vi "Stop Core.vi"(10 "final error code":i32, 11 "LF2R IDE in":refnum<class "Main Panel.lvclass">) -> (3 "LF2R IDE out":refnum<class "Main Panel.lvclass">)   [LabVIEW 2018, in "Main Panel.lvlib" / "Main Panel.lvclass"]
doc: "In addition to the following, this method also sends a message to the monitor to notify it that the actor has stopped execution.\n\n(<B>Filename</B>: Actor Framework.lvlib:Actor.lvclass:Stop Core.vi)\n\nDefines what the actor does before it stops. Use the <B>final error code</B> input to determine whether the actor shut down in response to an error.\n\nBy default, this method does nothing. A descendant class may override it to define behavior, such as shutting down any processes the actor initiated in its override of the Actor Core method.\n\nCopyright: MGI\n\nAuthored by Derek Trepanier\nsupport@mooregoodideas.com\nwww.mooregoodideas.com\n\nCopyright (c) 2014, Moore Good Ideas, Inc.\n\nAll rights reserved.\n\nRedistribution and use in source and binary forms, with or without modification, are permitted provided that the following conditions are met:\n\n * Redistributions of source code must retain the above copyright notice, this list of conditions and the following disclaimer.\n * Redistributions in binary form must reproduce the above copyright notice, this list of conditions and the following disclaimer in the documentation and/or other materials provided with the distribution.\n * Neither the name of Moore Good Ideas, Inc. nor the names of its contributors may be used to endorse or promote products derived from this software without specific prior written permission.\n\nTHIS SOFTWARE IS PROVIDED BY THE COPYRIGHT HOLDERS AND CONTRIBUTORS \"AS IS\" AND ANY EXPRESS OR IMPLIED WARRANTIES, INCLUDING, BUT NOT LIMITED TO, THE IMPLIED WARRANTIES OF MERCHANTABILITY AND FITNESS FOR A PARTICULAR PURPOSE ARE DISCLAIMED. IN NO EVENT SHALL THE COPYRIGHT OWNER OR CONTRIBUTORS BE LIABLE FOR ANY DIRECT, INDIRECT, INCIDENTAL, SPECIAL, EXEMPLARY, OR CONSEQUENTIAL DAMAGES (INCLUDING, BUT NOT LIMITED TO, PROCUREMENT OF SUBSTITUTE GOODS OR SERVICES; LOSS OF USE, DATA, OR PROFITS; OR BUSINESS INTERRUPTION) HOWEVER CAUSED AND ON ANY THEORY OF LIABILITY, WHETHER IN CONTRACT, STRICT LIABILITY, OR TORT (INCLUDING NEGLIGENCE OR OTHERWISE) ARISING IN ANY WAY OUT OF THE USE OF THIS SOFTWARE, EVEN IF ADVISED OF THE POSSIBILITY OF SUCH DAMAGE."
uses:
  Main Panel.lvclass
  Main Panel.lvclass/Main Panel.ctl
  Framework/Framework/Framework.lvclass
  <userlib>/_MGI/Menu Building/MenuTypes/Vi/MGI_VI.lvclass
  ScintillaNET/ScintillaNET.lvclass
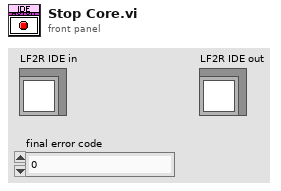
[diagram p1: front panel]
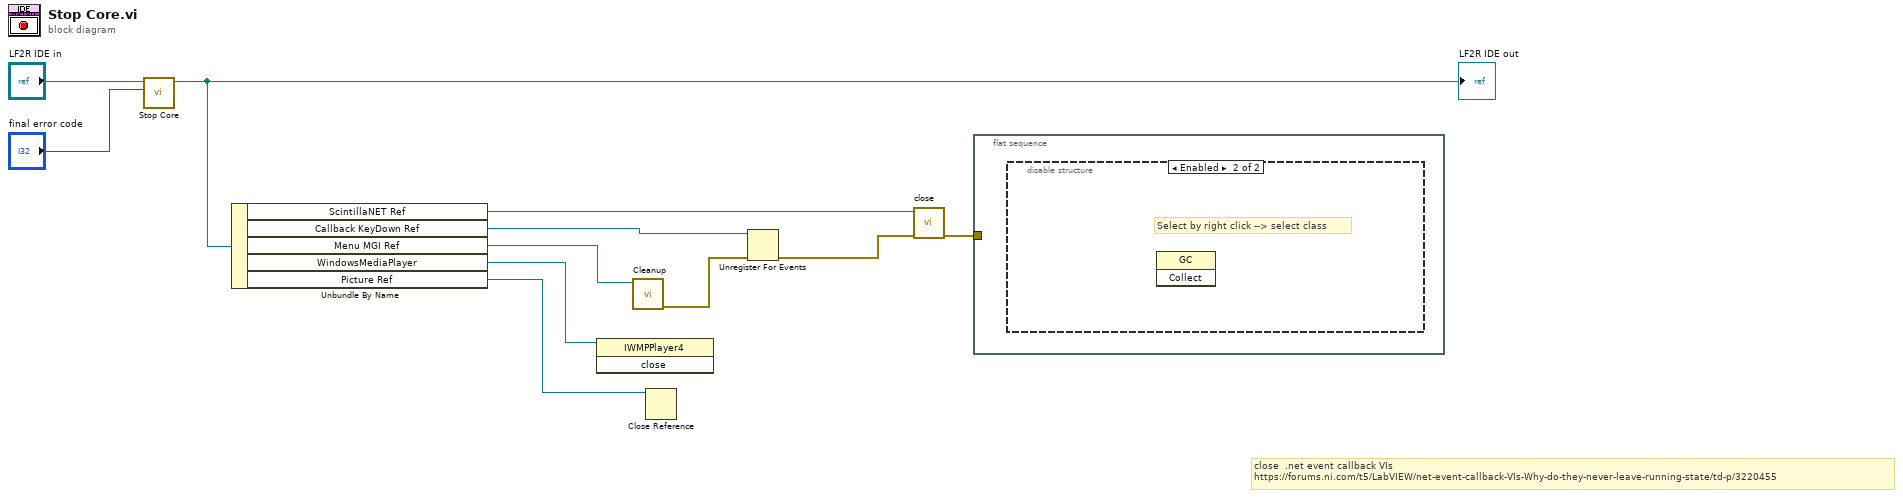
[diagram p0: block diagram]
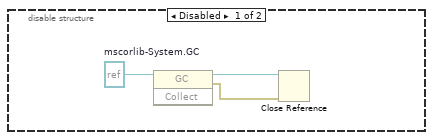
[diagram p2: hidden frame]
diagram:
  # "close  .net event callback VIs \nhttps://forums.ni.com/t5/LabVIEW/net-event-callback-VIs-Why-do-they-never-leave-running-state/td-p/3220455"
  n1 = call-parent "Stop Core.vi"("final error code"="final error code", "Monitored Actor in"="LF2R IDE in") -> ("Monitored Actor out"=w9:refnum<class "Main Panel.lvclass">)  [unwired: 9 in]
  "LF2R IDE out" <- w9
  n2 = Unbundle By Name(w9) -> ("ScintillaNET Ref"=w8:refnum<class "ScintillaNET.lvclass">, "Callback KeyDown Ref"=w6:refnum<k27>, "Menu MGI Ref"=w5:refnum<class "MGI_VI.lvclass">, "WindowsMediaPlayer"=w2:refnum<k7>, "Picture Ref"=w1:refnum<vi>)
  n3 = invoke class="IWMPPlayer4" method="close"(reference=w2) -> ()  [unwired: 2 in, 3 out]
  n4 = call-dynamic "Cleanup.vi"("VI"=w5) -> ("error out"=w3:errorcluster)  [unwired: 10 in]
  n5 = Close Reference(reference=w1) -> ()  [unwired: 1 in, 1 out]
  n6 = Unregister For Events(event registration refnum=w6, error in=w3) -> (error out=w7:errorcluster)
  n7 = call "close.vi"("error in (no error)"=w7, "ScintillaNET in"=w8) -> ("error out"=w4:errorcluster)  [unwired: 9 in]
  n8 = flat-sequence {
    tunnel: w4 -> [_]
    frame #0 {
      n9 = disable-structure shown="Enabled" {
        frame Disabled {
          w14 = refnum<k24> refnum  # mscorlib-System.GC
          n10 = invoke class="GC" method="Collect"(reference=w14) -> (reference out=w13:refnum<k24>, error out=w12:errorcluster)  [unwired: 2 in, 1 out]
          n11 = Close Reference(reference=w13, error in (no error)=w12) -> ()  [unwired: 1 out]
        }
        frame Enabled {
          # "Select by right click --> select class"
          n12 = invoke class="GC" method="Collect"() -> ()  [unwired: 3 in, 3 out]
        }
      }
    }
  }
